vi "svl_Integration Units.vi"(5 "desired base units for length":i32(ring) items=["no change"=-1, "m"=0, "mm"=2, "microns"=3, "in"=1, "mils"=5], 7 "integration type":T1(ring)=enum."double integration", 8 "error in (no error)":errorcluster, 11 "scaled signal [EU]":waveform(dbl)={"t0"=timestamp(0 s since 1904-01-01), "dt"=0.0, "Y"=[]}) -> (0 "error out":errorcluster, 2 "unit label":string, 3 "scaled signal out":waveform(dbl))   [LabVIEW 2017, in "SoundVib_Integration.lvlib"]
uses:
  <vilib>/addons/Sound and Vibration/svt_Integration/SoundVib_Integration.lvlib
  <vilib>/addons/_NISVFA/_Shared subVIs/Common/svc_Set SV Channel Info (variant).vi
  <vilib>/addons/_NISVFA/_Shared subVIs/Common/SVL Set dB Reference (variant).vi
  <vilib>/addons/_NISVFA/_Shared subVIs/Common/svc_Unit Label to Engineering Units.vi
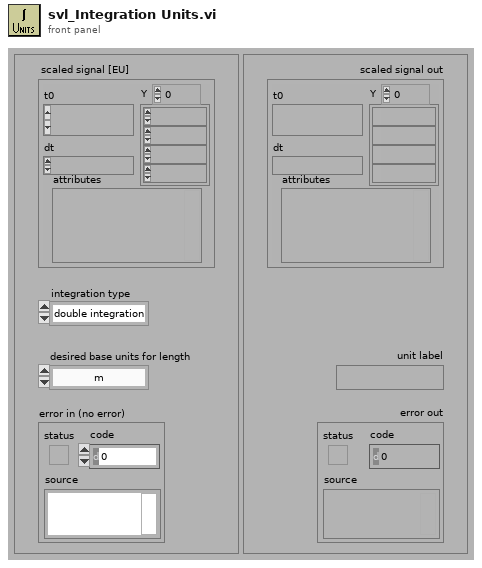
[diagram p1: front panel]
types:
  T1 = enum16{"single integration", "double integration"}
  T2 = typedef "svc_Channel Info.ctl" = cluster{"sensor sensitivity":dbl, "engineering units":T3, "dB reference":dbl, "custom label":string, "weighting filter":T4, "pregain":dbl}
  T3 = typedef "svc_Engineering Units Text Ring.ctl" = u16
  T4 = typedef "svc_Weighting Filter Text Ring.ctl" = u16
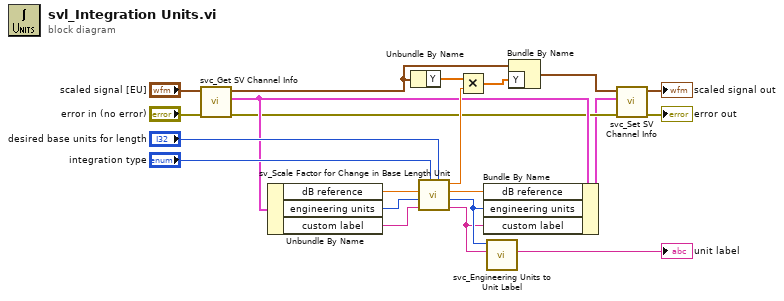
[diagram p0: block diagram]
diagram:
  n1 = call <vilib>:"svc_Get SV Channel Info.vi"("error in (no error)"="error in (no error)", "scaled signal [EU]"="scaled signal [EU]") -> ("error out"=w4:errorcluster, "channel info"=w6:T2, "dup scaled signal [EU]"=w12:waveform(dbl))  [unwired: 4 in, 3 out]
  n2 = Unbundle By Name(w6) -> ("dB reference"=w16:dbl, "engineering units"=w15:T3, "custom label"=w14:string)
  n3 = Unbundle By Name(w12) -> ("Y"=w8:dbl[])
  n4 = call <vilib>:"sv_Scale Factor for Change in Base Length Unit.vi"("desired base units for length"="desired base units for length", "integration type"="integration type", "custom label in"=w14, "engineering units in"=w15, "dB reference [EU] in"=w16) -> ("custom label out"=w13:string, "engineering units out"=w20:T3, "dB reference [EU] out"=w21:dbl, "units scale factor"=w7:dbl)  [unwired: 3 in]
  n5 = Multiply(x=w8, y=w7) -> (x*y=w5:dbl[])
  n6 = Bundle By Name(cluster=w6, "dB reference"=w21, "engineering units"=w20, "custom label"=w13) -> (w1:T2)
  n7 = call <vilib>:"svc_Engineering Units to Unit Label.vi"("custom label"=w13, "engineering units"=w20) -> ("unit label"=→"unit label":string)  [unwired: 8 in, 1 out]
  n8 = Bundle By Name(cluster=w12, "Y"=w5) -> (w11:waveform(dbl))
  n9 = call <vilib>:"svc_Set SV Channel Info.vi"("error in (no error)"=w4, "channel info"=w1, "scaled signal in"=w11) -> ("error out"=→"error out":errorcluster, "scaled signal out"=→"scaled signal out":waveform(dbl))  [unwired: 7 in]
